vi "GetDataClusters.vi"(11 "Data":variant) -> (0 "error out":errorcluster, 2 "Measurements":T1 {"Instrument Number" items=["1", "2", "3"]}, 3 "Device(s)Settings":T3={"MeasName"="", "Instr1"={"Name"="", "Vout (V)"=0.0, "VType"="", "FreqOut (Hz)"=60.0, "Aperture (cycles)"=1, "Synchronization"=0, "Ranges"={"Voltage (V)"=0, "Current (A)"=1}, "Safety Trips"={"Vmin (V)"=0.0, "Vmin Time (s)"=-1.0, "Vmax (V)"=0.0, "Vmax Time (s)"=-1.0, "Imax Source (A)"=0.0, "I Src Time (s)"=-1.0, "Imax Sink (A)"=0.0, "I Snk Time (s)"=-1.0, "Pmax Source (W)"=0.0, "P Src Time (s)"=-1.0, "Pmax Sink (W)"=0.0, "P Snk Time (s)"=-1.0, "Abs Volt Peak"=0.0, "Enable Vpk"=FALSE, "Abs Curr Peak"=0.0, "Enable Ipk"=FALSE}, "Slew Rates"={"Voltage (V/s)"=866030.0, "Current (A/s)"=100000.0, "Power (W/s)"=3000000.0, "Frequency (Hz/s)"=500.0, "Phase Angle (Deg/s)"=50000.0}, "Phases"={"A-Volts (V)"=0.0, "B-Volts (V)"=0.0, "C-Volts (V)"=0.0, "A-Change at..."=0, "B-Angle (Deg)"=240, "C-Angle (Deg)"=120, "B-Change at..."=0, "C-Change at..."=0, "AngleTxt"="", "A-Wave Shape"=0, "B-Wave Shape"=0, "C-Wave Shape"=0}}, "Instr2"={"Name"="", "Vout (V)"=0.0, "VType"="", "FreqOut (Hz)"=60.0, "Aperture (cycles)"=1, "Synchronization"=0, "Ranges"={"Voltage (V)"=0, "Current (A)"=1}, "Safety Trips"={"Vmin (V)"=0.0, "Vmin Time (s)"=-1.0, "Vmax (V)"=0.0, "Vmax Time (s)"=-1.0, "Imax Source (A)"=0.0, "I Src Time (s)"=-1.0, "Imax Sink (A)"=0.0, "I Snk Time (s)"=-1.0, "Pmax Source (W)"=0.0, "P Src Time (s)"=-1.0, "Pmax Sink (W)"=0.0, "P Snk Time (s)"=-1.0, "Abs Volt Peak"=0.0, "Enable Vpk"=FALSE, "Abs Curr Peak"=0.0, "Enable Ipk"=FALSE}, "Slew Rates"={"Voltage (V/s)"=866030.0, "Current (A/s)"=100000.0, "Power (W/s)"=3000000.0, "Frequency (Hz/s)"=500.0, "Phase Angle (Deg/s)"=50000.0}, "Phases"={"A-Volts (V)"=0.0, "B-Volts (V)"=0.0, "C-Volts (V)"=0.0, "A-Change at..."=0, "B-Angle (Deg)"=240, "C-Angle (Deg)"=120, "B-Change at..."=0, "C-Change at..."=0, "AngleTxt"="", "A-Wave Shape"=0, "B-Wave Shape"=0, "C-Wave Shape"=0}}, "Instr3"={"Name"="", "Vout (V)"=0.0, "VType"="", "FreqOut (Hz)"=60.0, "Aperture (cycles)"=1, "Synchronization"=0, "Ranges"={"Voltage (V)"=0, "Current (A)"=1}, "Safety Trips"={"Vmin (V)"=0.0, "Vmin Time (s)"=-1.0, "Vmax (V)"=0.0, "Vmax Time (s)"=-1.0, "Imax Source (A)"=0.0, "I Src Time (s)"=-1.0, "Imax Sink (A)"=0.0, "I Snk Time (s)"=-1.0, "Pmax Source (W)"=0.0, "P Src Time (s)"=-1.0, "Pmax Sink (W)"=0.0, "P Snk Time (s)"=-1.0, "Abs Volt Peak"=0.0, "Enable Vpk"=FALSE, "Abs Curr Peak"=0.0, "Enable Ipk"=FALSE}, "Slew Rates"={"Voltage (V/s)"=866030.0, "Current (A/s)"=100000.0, "Power (W/s)"=3000000.0, "Frequency (Hz/s)"=500.0, "Phase Angle (Deg/s)"=50000.0}, "Phases"={"A-Volts (V)"=0.0, "B-Volts (V)"=0.0, "C-Volts (V)"=0.0, "A-Change at..."=0, "B-Angle (Deg)"=240, "C-Angle (Deg)"=120, "B-Change at..."=0, "C-Change at..."=0, "AngleTxt"="", "A-Wave Shape"=0, "B-Wave Shape"=0, "C-Wave Shape"=0}}, "Handle"="", "Reset"=FALSE, "Mode"=0, "ID Query"=FALSE, "Connected"=FALSE, "Chassis"=1, "VRangeVals1"=[], "SyncList1"=[], "Wave1A"=[], "Wave1B"=[], "Wave1C"=[], "SyncList2"=[], "SyncList3"=[], "VRangeVals3"=[], "VRangeVals2"=[], "CRangeVals1"=[], "CRangeVals3"=[], "CRangeVals2"=[], "TabPages"=[], "Wave2A"=[], "Wave2B"=[], "Wave2C"=[], "Wave3A"=[], "Wave3B"=[], "Wave3C"=[], "EnableCtrls"=[[1, 0, 0, 0, 0, 0, 0, 0, 0, 0, 0, 0, 0, 0, 0, 0, 0, 0], [1, 0, 0, 0, 0, 0, 0, 0, 0, 0, 0, 0, 0, 0, 0, 0, 0, 0], [1, 0, 0, 0, 0, 0, 0, 0, 0, 0, 0, 0, 0, 0, 0, 0, 0, 0]]} {"Chassis" min=1 max=8 step=1; "Mode" items=["3-Phase AC"=0, "AC"=1, "DC"=2, "AC - AC"=7, "AC - DC"=8, "DC - AC"=11, "DC - DC"=12, "2-Phase AC - AC"=5, "2-Phase AC - DC"=6, "AC - AC - AC"=3, "DC - DC - DC"=4, "AC - AC - DC"=9, "AC - DC - DC"=10, "AC - DC - AC"=13, "DC - AC - AC"=14, "DC - AC - DC"=15]; "Instr3"."Phases"."C-Wave Shape" items=["Sine", "User1", "User2", "User3"]; "Instr3"."Phases"."B-Wave Shape" items=["Sine", "User1", "User2", "User3"]; "Instr3"."Phases"."A-Wave Shape" items=["Sine", "User1", "User2", "User3"]; "Instr3"."Phases"."C-Change at..." min=0 max=359; "Instr3"."Phases"."B-Change at..." min=0 max=359; "Instr3"."Phases"."A-Change at..." min=0 max=359; "Instr3"."Phases"."C-Angle (Deg)" min=0 max=359; "Instr3"."Phases"."B-Angle (Deg)" min=0 max=359; "Instr3"."Phases"."C-Volts (V)" min=0.0 max=606.0; "Instr3"."Phases"."B-Volts (V)" min=0.0 max=606.0; "Instr3"."Phases"."A-Volts (V)" min=0.0 max=606.0; "Instr3"."Slew Rates"."Phase Angle (Deg/s)" min=0.1 max=50000.0; "Instr3"."Slew Rates"."Frequency (Hz/s)" min=0.01 max=500.0; "Instr3"."Slew Rates"."Power (W/s)" min=2.0 max=8000000.0; "Instr3"."Slew Rates"."Current (A/s)" min=0.2 max=2400000.0; "Instr3"."Slew Rates"."Voltage (V/s)" min=0.01 max=2000000.0; "Instr3"."Safety Trips"."Abs Curr Peak" min=0.0; "Instr3"."Safety Trips"."Abs Volt Peak" min=0.0; "Instr3"."Safety Trips"."P Snk Time (s)" min=-1.0 max=3600.0; "Instr3"."Safety Trips"."Pmax Sink (W)" min=0.0 max=436000.0 format="%#_7g"; "Instr3"."Safety Trips"."P Src Time (s)" min=-1.0 max=3600.0; "Instr3"."Safety Trips"."Pmax Source (W)" min=0.0 max=436000.0 format="%#_7g"; "Instr3"."Safety Trips"."I Snk Time (s)" min=-1.0 max=3600.0; "Instr3"."Safety Trips"."Imax Sink (A)" min=0.0 max=720.0; "Instr3"."Safety Trips"."I Src Time (s)" min=-1.0 max=3600.0; "Instr3"."Safety Trips"."Imax Source (A)" min=0.0 max=720.0; "Instr3"."Safety Trips"."Vmax Time (s)" min=-1.0 max=3600.0; "Instr3"."Safety Trips"."Vmax (V)" min=0.0 max=606.0; "Instr3"."Safety Trips"."Vmin Time (s)" min=-1.0 max=3600.0; "Instr3"."Safety Trips"."Vmin (V)" min=0.0 max=606.0; "Instr3"."Ranges"."Current (A)" items=["6", "30"]; "Instr3"."Ranges"."Voltage (V)" items=["303", "606"]; "Instr3"."Synchronization" items=["Immediate", "Sync to Phase A"]; "Instr3"."Aperture (cycles)" min=0 max=64; "Instr3"."FreqOut (Hz)" min=30.0 max=880.0; "Instr3"."Vout (V)" min=0.0 max=606.0; "Instr2"."Phases"."C-Wave Shape" items=["Sine", "User1", "User2", "User3"]; "Instr2"."Phases"."B-Wave Shape" items=["Sine", "User1", "User2", "User3"]; "Instr2"."Phases"."A-Wave Shape" items=["Sine", "User1", "User2", "User3"]; "Instr2"."Phases"."C-Change at..." min=0 max=359; "Instr2"."Phases"."B-Change at..." min=0 max=359; "Instr2"."Phases"."A-Change at..." min=0 max=359; "Instr2"."Phases"."C-Angle (Deg)" min=0 max=359; "Instr2"."Phases"."B-Angle (Deg)" min=0 max=359; "Instr2"."Phases"."C-Volts (V)" min=0.0 max=606.0; "Instr2"."Phases"."B-Volts (V)" min=0.0 max=606.0; "Instr2"."Phases"."A-Volts (V)" min=0.0 max=606.0; "Instr2"."Slew Rates"."Phase Angle (Deg/s)" min=0.1 max=50000.0; "Instr2"."Slew Rates"."Frequency (Hz/s)" min=0.01 max=500.0; "Instr2"."Slew Rates"."Power (W/s)" min=2.0 max=8000000.0; "Instr2"."Slew Rates"."Current (A/s)" min=0.2 max=2400000.0; "Instr2"."Slew Rates"."Voltage (V/s)" min=0.01 max=2000000.0; "Instr2"."Safety Trips"."Abs Curr Peak" min=0.0; "Instr2"."Safety Trips"."Abs Volt Peak" min=0.0; "Instr2"."Safety Trips"."P Snk Time (s)" min=-1.0 max=3600.0; "Instr2"."Safety Trips"."Pmax Sink (W)" min=0.0 max=436000.0 format="%#_7g"; "Instr2"."Safety Trips"."P Src Time (s)" min=-1.0 max=3600.0; "Instr2"."Safety Trips"."Pmax Source (W)" min=0.0 max=436000.0 format="%#_7g"; "Instr2"."Safety Trips"."I Snk Time (s)" min=-1.0 max=3600.0; "Instr2"."Safety Trips"."Imax Sink (A)" min=0.0 max=720.0; "Instr2"."Safety Trips"."I Src Time (s)" min=-1.0 max=3600.0; "Instr2"."Safety Trips"."Imax Source (A)" min=0.0 max=720.0; "Instr2"."Safety Trips"."Vmax Time (s)" min=-1.0 max=3600.0; "Instr2"."Safety Trips"."Vmax (V)" min=0.0 max=606.0; "Instr2"."Safety Trips"."Vmin Time (s)" min=-1.0 max=3600.0; "Instr2"."Safety Trips"."Vmin (V)" min=0.0 max=606.0; "Instr2"."Ranges"."Current (A)" items=["6", "30"]; "Instr2"."Ranges"."Voltage (V)" items=["303", "606"]; "Instr2"."Synchronization" items=["Immediate", "Sync to Phase A"]; "Instr2"."Aperture (cycles)" min=0 max=64; "Instr2"."FreqOut (Hz)" min=30.0 max=880.0; "Instr2"."Vout (V)" min=0.0 max=606.0; "Instr1"."Phases"."C-Wave Shape" items=["Sine", "User1", "User2", "User3"]; "Instr1"."Phases"."B-Wave Shape" items=["Sine", "User1", "User2", "User3"]; "Instr1"."Phases"."A-Wave Shape" items=["Sine", "User1", "User2", "User3"]; "Instr1"."Phases"."C-Change at..." min=0 max=359; "Instr1"."Phases"."B-Change at..." min=0 max=359; "Instr1"."Phases"."A-Change at..." min=0 max=359; "Instr1"."Phases"."C-Angle (Deg)" min=0 max=359; "Instr1"."Phases"."B-Angle (Deg)" min=0 max=359; "Instr1"."Phases"."C-Volts (V)" min=0.0 max=606.0; "Instr1"."Phases"."B-Volts (V)" min=0.0 max=606.0; "Instr1"."Phases"."A-Volts (V)" min=0.0 max=606.0; "Instr1"."Slew Rates"."Phase Angle (Deg/s)" min=0.1 max=50000.0; "Instr1"."Slew Rates"."Frequency (Hz/s)" min=0.01 max=500.0; "Instr1"."Slew Rates"."Power (W/s)" min=2.0 max=8000000.0; "Instr1"."Slew Rates"."Current (A/s)" min=0.2 max=2400000.0; "Instr1"."Slew Rates"."Voltage (V/s)" min=0.01 max=2000000.0; "Instr1"."Safety Trips"."Abs Curr Peak" min=0.0; "Instr1"."Safety Trips"."Abs Volt Peak" min=0.0; "Instr1"."Safety Trips"."P Snk Time (s)" min=-1.0 max=3600.0; "Instr1"."Safety Trips"."Pmax Sink (W)" min=0.0 max=436000.0 format="%#_7g"; "Instr1"."Safety Trips"."P Src Time (s)" min=-1.0 max=3600.0; "Instr1"."Safety Trips"."Pmax Source (W)" min=0.0 max=436000.0 format="%#_7g"; "Instr1"."Safety Trips"."I Snk Time (s)" min=-1.0 max=3600.0; "Instr1"."Safety Trips"."Imax Sink (A)" min=0.0 max=720.0; "Instr1"."Safety Trips"."I Src Time (s)" min=-1.0 max=3600.0; "Instr1"."Safety Trips"."Imax Source (A)" min=0.0 max=720.0; "Instr1"."Safety Trips"."Vmax Time (s)" min=-1.0 max=3600.0; "Instr1"."Safety Trips"."Vmax (V)" min=0.0 max=606.0; "Instr1"."Safety Trips"."Vmin Time (s)" min=-1.0 max=3600.0; "Instr1"."Safety Trips"."Vmin (V)" min=0.0 max=606.0; "Instr1"."Ranges"."Current (A)" items=["6", "30"]; "Instr1"."Ranges"."Voltage (V)" items=["303", "606"]; "Instr1"."Synchronization" items=["Immediate", "Sync to Phase A"]; "Instr1"."Aperture (cycles)" min=0 max=64; "Instr1"."FreqOut (Hz)" min=30.0 max=880.0; "Instr1"."Vout (V)" min=0.0 max=606.0})   [LabVIEW 2018, in "Visualization.lvlib" / "VisualizeAcPwr.lvclass"]
doc: "This VI is used only to reduce the length of the labels for the 'unbundle-by-name' elements coming out of the Variant-to-Data block if it was used directly."
uses:
  VisualizeAcPwr.lvclass
  AcPwr/AcPwrPlugins/NHRGridSimClass/TypeDefs/Device(s)Settings.ctl
  AcPwr/AcPwrPlugins/NHRGridSimClass/TypeDefs/NHRGrid_InstrumentCluster_Tabs.ctl
  AcPwr/AcPwrPlugins/NHRGridSimClass/TypeDefs/NHRGrid_Configure_Tabs.ctl
  AcPwr/AcPwrPlugins/NHRGridSimClass/TypeDefs/NHRGrid_Ranges_Tabs.ctl
  AcPwr/AcPwrPlugins/NHRGridSimClass/TypeDefs/NHRGrid_SafetyTrips_Tabs.ctl
  AcPwr/AcPwrPlugins/NHRGridSimClass/TypeDefs/NHRGrid_SlewRates_Tabs.ctl
  AcPwr/AcPwrPlugins/NHRGridSimClass/TypeDefs/NHRGrid_Phases_Tabs.ctl
  AcPwr/AcPwrPlugins/NHRGridSimClass/TypeDefs/NHRGrid_Modes.ctl
  AcPwr/AcPwrPlugins/NHRGridSimClass/PublicMethods/Measurements.ctl
  AcPwr/AcPwrPlugins/NHRGridSimClass/TypeDefs/MeasurementType.ctl
  AcPwr/AcPwrPlugins/NHRGridSimClass/TypeDefs/DeviceConfig&Meas.ctl
  AcPwr/AcPwrPlugins/NHRGridSimClass/NHRGridSim.lvclass
panel:
  # "Row = Instrument\nColumn: 0-Name, 1-FreqOut, 2-Sync, 3-AVolts, 4-BVolts, 5-CVolts, 6-BAngle, 7-CAngle, 8-AChange, 9-BChange, 10-CChange, 11-AWave, 12-BWave, 13-CWave, 14-SlewCurr, 15-SlewPower, 16-SlewFreq, 17-SlewPhase"
  # "0= Enabled, 1= Disabled, 2= Disabled and Greyed"
  # "Degrees with Respect to Phase A"
  # "Voltages (L-N)"
  # "Degrees for Synchronization"
  # "AC Phase Waveform"
  # "Degrees with Respect to Phase A"
  # "Voltages (L-N)"
  # "Degrees for Synchronization"
  # "AC Phase Waveform"
  # "Degrees with Respect to Phase A"
  # "Voltages (L-N)"
  # "Degrees for Synchronization"
  # "AC Phase Waveform"
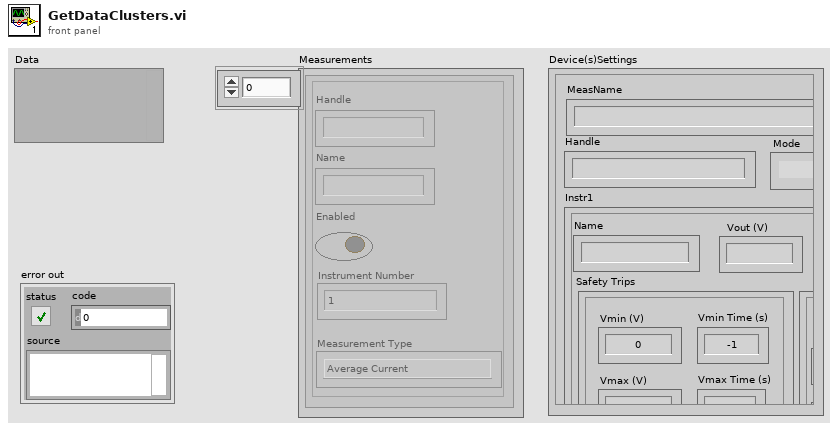
[diagram p1: front panel]
types:
  T1 = typedef "AcPwrPlugins.lvlib/NHRGridSim.lvclass/Measurements.ctl" = cluster{"Handle":string, "Name":string, "Enabled ":bool, "Measurement Value":dbl, "Instrument Number ":i32, "Measurement Type ":T2}[]
  T2 = typedef "AcPwrPlugins.lvlib/NHRGridSim.lvclass/MeasurementType.ctl" = enum16{"Average Current", "Average Voltage"}
  T3 = typedef "AcPwrPlugins.lvlib/NHRGridSim.lvclass/Device(s)Settings.ctl" = cluster{"MeasName":string, "Instr1":T4, "Instr2":T4, "Instr3":T4, "Handle":string, "Reset":bool, "Mode":T10, "ID Query":bool, "Connected":bool, "Chassis":i32, "VRangeVals1":string[], "SyncList1":string[], "Wave1A":string[], "Wave1B":string[], "Wave1C":string[], "SyncList2":string[], "SyncList3":string[], "VRangeVals3":string[], "VRangeVals2":string[], "CRangeVals1":string[], "CRangeVals3":string[], "CRangeVals2":string[], "TabPages":bool[], "Wave2A":string[], "Wave2B":string[], "Wave2C":string[], "Wave3A":string[], "Wave3B":string[], "Wave3C":string[], "EnableCtrls":i8[][]}
  T4 = typedef "AcPwrPlugins.lvlib/NHRGridSim.lvclass/NHRGrid_InstrumentCluster_Tabs.ctl" = cluster{"Name":string, "Vout (V)":dbl, "VType":string, "FreqOut (Hz)":dbl, "Aperture (cycles)":i32, "Synchronization":T5, "Ranges":T6, "Safety Trips":T7, "Slew Rates":T8, "Phases":T9}
  T5 = typedef "AcPwrPlugins.lvlib/NHRGridSim.lvclass/NHRGrid_Configure_Tabs.ctl" = u16
  T6 = typedef "AcPwrPlugins.lvlib/NHRGridSim.lvclass/NHRGrid_Ranges_Tabs.ctl" = cluster{"Voltage (V)":u16, "Current (A)":u16}
  T7 = typedef "AcPwrPlugins.lvlib/NHRGridSim.lvclass/NHRGrid_SafetyTrips_Tabs.ctl" = cluster{"Vmin (V)":dbl, "Vmin Time (s)":dbl, "Vmax (V)":dbl, "Vmax Time (s)":dbl, "Imax Source (A)":dbl, "I Src Time (s)":dbl, "Imax Sink (A)":dbl, "I Snk Time (s)":dbl, "Pmax Source (W)":dbl, "P Src Time (s)":dbl, "Pmax Sink (W)":dbl, "P Snk Time (s)":dbl, "Abs Volt Peak":dbl, "Enable Vpk":bool, "Abs Curr Peak":dbl, "Enable Ipk":bool}
  T8 = typedef "AcPwrPlugins.lvlib/NHRGridSim.lvclass/NHRGrid_SlewRates_Tabs.ctl" = cluster{"Voltage (V/s)":dbl, "Current (A/s)":dbl, "Power (W/s)":dbl, "Frequency (Hz/s)":dbl, "Phase Angle (Deg/s)":dbl}
  T9 = typedef "AcPwrPlugins.lvlib/NHRGridSim.lvclass/NHRGrid_Phases_Tabs.ctl" = cluster{"A-Volts (V)":dbl, "B-Volts (V)":dbl, "C-Volts (V)":dbl, "A-Change at...":i32, "B-Angle (Deg)":i32, "C-Angle (Deg)":i32, "B-Change at...":i32, "C-Change at...":i32, "AngleTxt":string, "A-Wave Shape":u16, "B-Wave Shape":u16, "C-Wave Shape":u16}
  T10 = typedef "AcPwrPlugins.lvlib/NHRGridSim.lvclass/NHRGrid_Modes.ctl" = u8
  T11 = typedef "AcPwrPlugins.lvlib/NHRGridSim.lvclass/DeviceConfig&Meas.ctl" = cluster{"Device(s)Settings":T3, "Measurements":T1}
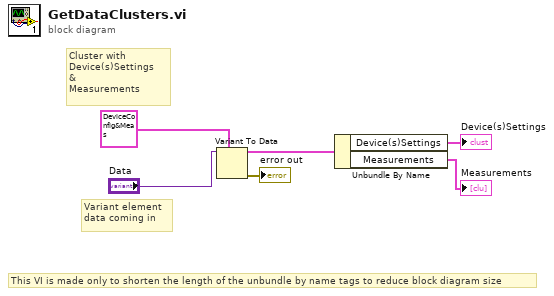
[diagram p0: block diagram]
diagram:
  # "This VI is made only to shorten the length of the unbundle by name tags to reduce block diagram size"
  # "Cluster with Device(s)Settings\n&\nMeasurements"
  # "Variant element data coming in"
  n1 = Variant To Data(type=T11 {"Device(s)Settings"={"MeasName"="", "Instr1"={"Name"="", "Vout (V)"=0.0, "VType"="", "FreqOut (Hz)"=0.0, "Aperture (cycles)"=0, "Synchronization"=0, "Ranges"={"Voltage (V)"=0, "Current (A)"=0}, "Safety Trips"={"Vmin (V)"=0.0, "Vmin Time (s)"=0.0, "Vmax (V)"=0.0, "Vmax Time (s)"=0.0, "Imax Source (A)"=0.0, "I Src Time (s)"=0.0, "Imax Sink (A)"=0.0, "I Snk Time (s)"=0.0, "Pmax Source (W)"=0.0, "P Src Time (s)"=0.0, "Pmax Sink (W)"=0.0, "P Snk Time (s)"=0.0, "Abs Volt Peak"=0.0, "Enable Vpk"=FALSE, "Abs Curr Peak"=0.0, "Enable Ipk"=FALSE}, "Slew Rates"={"Voltage (V/s)"=0.0, "Current (A/s)"=0.0, "Power (W/s)"=0.0, "Frequency (Hz/s)"=0.0, "Phase Angle (Deg/s)"=0.0}, "Phases"={"A-Volts (V)"=0.0, "B-Volts (V)"=0.0, "C-Volts (V)"=0.0, "A-Change at..."=0, "B-Angle (Deg)"=0, "C-Angle (Deg)"=0, "B-Change at..."=0, "C-Change at..."=0, "AngleTxt"="", "A-Wave Shape"=0, "B-Wave Shape"=0, "C-Wave Shape"=0}}, "Instr2"={"Name"="", "Vout (V)"=0.0, "VType"="", "FreqOut (Hz)"=0.0, "Aperture (cycles)"=0, "Synchronization"=0, "Ranges"={"Voltage (V)"=0, "Current (A)"=0}, "Safety Trips"={"Vmin (V)"=0.0, "Vmin Time (s)"=0.0, "Vmax (V)"=0.0, "Vmax Time (s)"=0.0, "Imax Source (A)"=0.0, "I Src Time (s)"=0.0, "Imax Sink (A)"=0.0, "I Snk Time (s)"=0.0, "Pmax Source (W)"=0.0, "P Src Time (s)"=0.0, "Pmax Sink (W)"=0.0, "P Snk Time (s)"=0.0, "Abs Volt Peak"=0.0, "Enable Vpk"=FALSE, "Abs Curr Peak"=0.0, "Enable Ipk"=FALSE}, "Slew Rates"={"Voltage (V/s)"=0.0, "Current (A/s)"=0.0, "Power (W/s)"=0.0, "Frequency (Hz/s)"=0.0, "Phase Angle (Deg/s)"=0.0}, "Phases"={"A-Volts (V)"=0.0, "B-Volts (V)"=0.0, "C-Volts (V)"=0.0, "A-Change at..."=0, "B-Angle (Deg)"=0, "C-Angle (Deg)"=0, "B-Change at..."=0, "C-Change at..."=0, "AngleTxt"="", "A-Wave Shape"=0, "B-Wave Shape"=0, "C-Wave Shape"=0}}, "Instr3"={"Name"="", "Vout (V)"=0.0, "VType"="", "FreqOut (Hz)"=0.0, "Aperture (cycles)"=0, "Synchronization"=0, "Ranges"={"Voltage (V)"=0, "Current (A)"=0}, "Safety Trips"={"Vmin (V)"=0.0, "Vmin Time (s)"=0.0, "Vmax (V)"=0.0, "Vmax Time (s)"=0.0, "Imax Source (A)"=0.0, "I Src Time (s)"=0.0, "Imax Sink (A)"=0.0, "I Snk Time (s)"=0.0, "Pmax Source (W)"=0.0, "P Src Time (s)"=0.0, "Pmax Sink (W)"=0.0, "P Snk Time (s)"=0.0, "Abs Volt Peak"=0.0, "Enable Vpk"=FALSE, "Abs Curr Peak"=0.0, "Enable Ipk"=FALSE}, "Slew Rates"={"Voltage (V/s)"=0.0, "Current (A/s)"=0.0, "Power (W/s)"=0.0, "Frequency (Hz/s)"=0.0, "Phase Angle (Deg/s)"=0.0}, "Phases"={"A-Volts (V)"=0.0, "B-Volts (V)"=0.0, "C-Volts (V)"=0.0, "A-Change at..."=0, "B-Angle (Deg)"=0, "C-Angle (Deg)"=0, "B-Change at..."=0, "C-Change at..."=0, "AngleTxt"="", "A-Wave Shape"=0, "B-Wave Shape"=0, "C-Wave Shape"=0}}, "Handle"="", "Reset"=FALSE, "Mode"=0, "ID Query"=FALSE, "Connected"=FALSE, "Chassis"=0, "VRangeVals1"=[], "SyncList1"=[], "Wave1A"=[], "Wave1B"=[], "Wave1C"=[], "SyncList2"=[], "SyncList3"=[], "VRangeVals3"=[], "VRangeVals2"=[], "CRangeVals1"=[], "CRangeVals3"=[], "CRangeVals2"=[], "TabPages"=[], "Wave2A"=[], "Wave2B"=[], "Wave2C"=[], "Wave3A"=[], "Wave3B"=[], "Wave3C"=[], "EnableCtrls"=[]}, "Measurements"=[]} ("output cluster"), Variant="Data") -> (data=w4:T11, error out=→"error out":errorcluster)  [unwired: 1 in]
  n2 = Unbundle By Name(w4) -> ("Device(s)Settings"=→"Device(s)Settings":T3, "Measurements"=→"Measurements":T1)
